vi "NF LI56xx dvr qFETCh.vi"(8 "error in":errorcluster caption="error in (no error)" {"code" format="%.0x"}, 11 "VISA resource name":refnum<visa-resource-name>) -> (0 "error out":errorcluster {"code" format="%.0x"}, 2 "measurement data":string, 3 "VISA resource name copy":refnum<visa-resource-name>)   [LabVIEW 2019]
doc: "Queries the most recent measurement data."
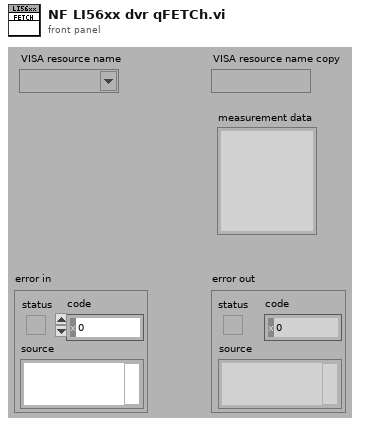
[diagram p1: front panel]
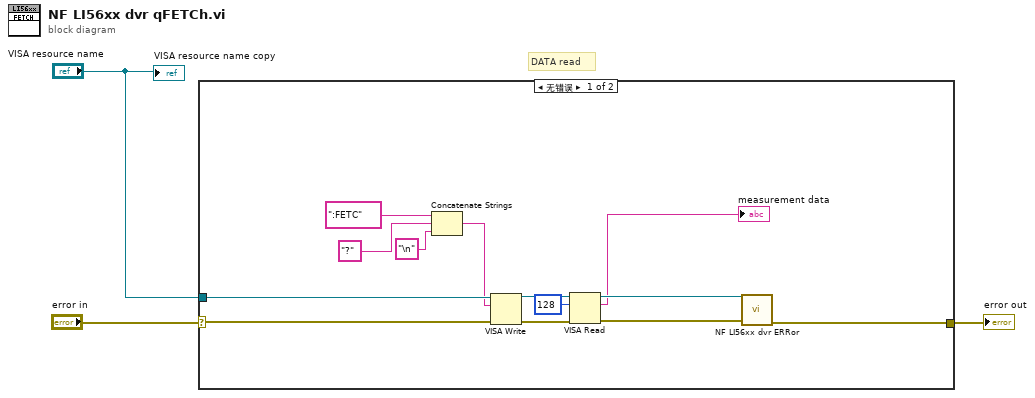
[diagram p0: block diagram]
diagram:
  # "DATA read"
  n1 = case shown="无错误" "error in" {
    selector: "error in" -> [w16 w17]
    tunnel: [w14 w17] -> w3
    tunnel: "VISA resource name" -> [w15 _]
    frame No Error {
      n2 = Concatenate Strings(":FETC" ("•¶Žš—ñ"), "?" ("Œ`Ž®•¶Žš—ñ"), "\n" ("Œ`Ž®•¶Žš—ñ")) -> (w13:string)
      n3 = VISA Write(VISA resource name=w15, write buffer=w13, error in (no error)=w16) -> (VISA resource name out=w10:refnum<visa-resource-name>, error out=w8:errorcluster)  [unwired: 1 out]
      n4 = VISA Read(VISA resource name=w10, byte count=u32 128 ("バイトカウント（0）"), error in (no error)=w8) -> (VISA resource name out=w9:refnum<visa-resource-name>, read buffer=→"measurement data":string, error out=w7:errorcluster)  [unwired: 1 out]
      n5 = call "NF LI56xx dvr ERRor.vi"("VISA resource name"=w9, "error in (no error)"=w7) -> ("error out"=w14:errorcluster)  [unwired: 10 in, 3 out]
    }
    frame Error {
    }
  }
  "error out" <- w3
  "VISA resource name copy" <- "VISA resource name"
